vi "AlazarGetStatus.vi"(0 "Handle":u64, 5 "error in (no error)":errorcluster) -> (14 "Handle":u64, 15 "Trig. Timeout":bool, 16 "Chan. A out of range":bool, 17 "Chan. B out of range":bool, 18 "PLL Locked":bool, 19 "error out":errorcluster)   [LabVIEW 2018]
doc: "Return a bitmask with board status information."
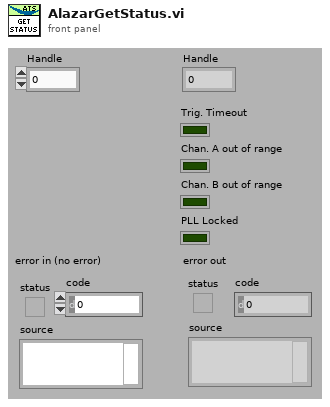
[diagram p1: front panel]
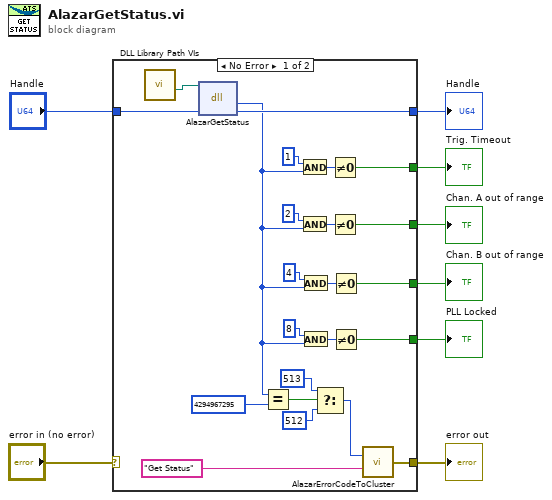
[diagram p0: block diagram]
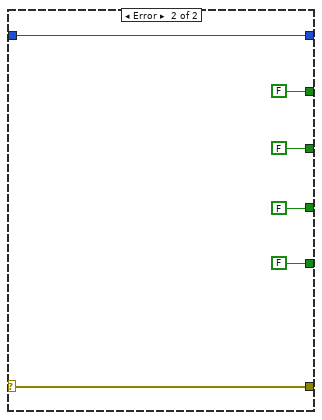
[diagram p2: hidden frame]
diagram:
  n1 = case shown="No Error" "error in (no error)" {
    selector: "error in (no error)" -> [_ w37]
    tunnel: [w29 w37] -> w7
    tunnel: "Handle" -> [w31 w36]
    tunnel: [w28 w36] -> w5
    tunnel: [w13 FALSE] -> w4
    tunnel: [w12 FALSE] -> w3
    tunnel: [w11 FALSE] -> w2
    tunnel: [w10 FALSE] -> w1
    frame No Error {
      n2 = call "DLL Library Path VIs.vi"() -> ("Alazar"=w9:path)  [unwired: 9 in, 2 out]
      n3 = dll-call lib="C:/Project/SerialSectOCT - FFT GPU/SerialSectOCT/Labview Software/DLL/ATSApi.dll" fn="AlazarGetStatus"(path in=w9, "handle"=w31) -> ("return type"=w14:u32, "handle"=w28:u64)  [unwired: 2 in, 2 out]
      n4 = Equal?(x=w14, y=u32 4294967295) -> (x = y?=w26:bool)
      n5 = And(x=u32 1, y=w14) -> (x .and. y?=w21:u32)
      n6 = And(x=u32 2, y=w14) -> (x .and. y?=w19:u32)
      n7 = And(x=u32 4, y=w14) -> (x .and. y?=w17:u32)
      n8 = And(x=u32 8, y=w14) -> (x .and. y?=w15:u32)
      n9 = Select(t=u32 513, s=w26, f=u32 512) -> (s? t:f=w23:u32)
      n10 = Not Equal To 0?(x=w21) -> (x != 0?=w13:bool)
      n11 = Not Equal To 0?(x=w19) -> (x != 0?=w12:bool)
      n12 = Not Equal To 0?(x=w17) -> (x != 0?=w11:bool)
      n13 = Not Equal To 0?(x=w15) -> (x != 0?=w10:bool)
      n14 = call "AlazarErrorCodeToCluster.vi"("Message"="Get Status", "Error Code"=w23) -> ("error out"=w29:errorcluster)
    }
    frame Error {
    }
  }
  "Handle" <- w5
  "error out" <- w7
  "Chan. B out of range" <- w2
  "PLL Locked" <- w1
  "Chan. A out of range" <- w3
  "Trig. Timeout" <- w4
